vi "对称性单.vi"(11 "XY图":cluster{dbl[], dbl[]}[](graph)) -> (3 "对称性":dbl)   [LabVIEW 2020]
uses:
  <vilib>/Analysis/NI_AAL_Geometry.lvlib
panel:
  out "右":dbl
  out "左":dbl
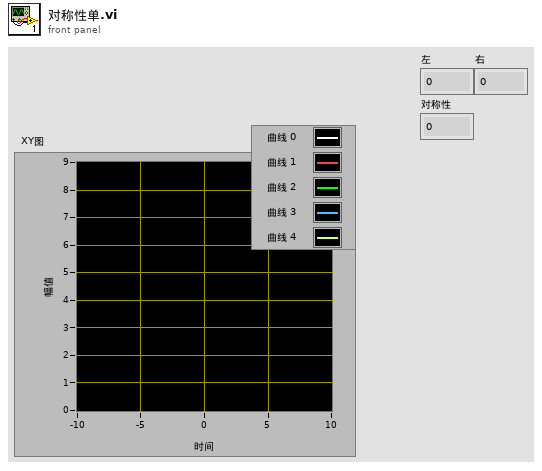
[diagram p1: front panel]
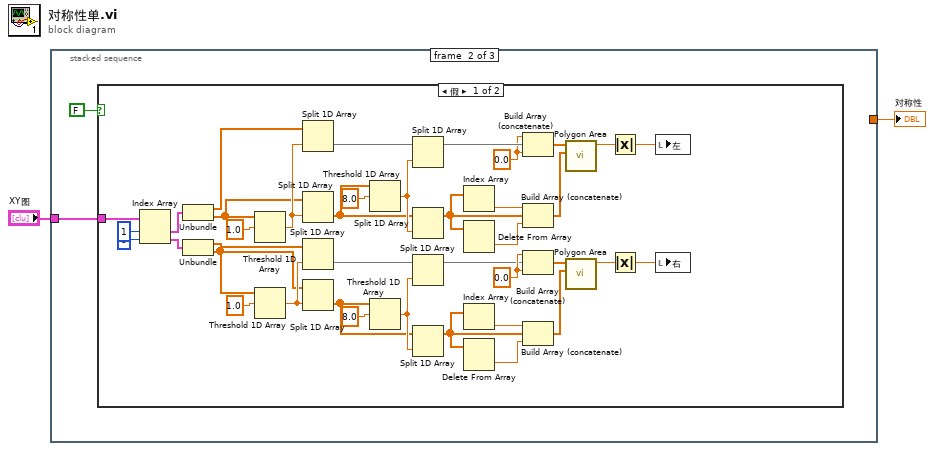
[diagram p0: block diagram]
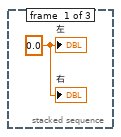
[diagram p2: hidden frame]
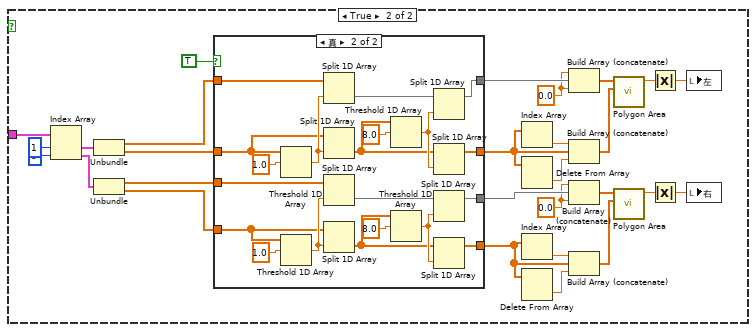
[diagram p3: hidden frame]
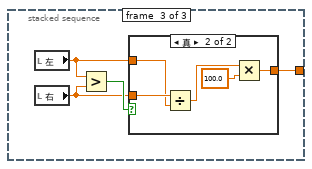
[diagram p5: hidden frame]
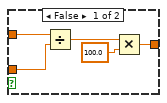
[diagram p6: hidden frame]
diagram:
  n1 = stacked-sequence {
    tunnel: "XY图" -> [_ w4 _]
    tunnel: [_ _ w97] -> w2
    frame #0 {
      w3 = 0.0 ("左")
      "左" <- w3
      "右" <- w3
    }
    frame #1 {
      n2 = case shown="假" FALSE {
        tunnel: w4 -> [w39 w49]
        frame False {
          w13 = 0.0
          w21 = 0.0
          n3 = Index Array(array=w39, index #1=1 ("索引"), index #2=3 ("索引")) -> (element #1=w40:cluster{dbl[], dbl[]}, element #2=w8:cluster{dbl[], dbl[]})
          n4 = Unbundle(w40) -> (w37:dbl[], w31:dbl[])
          n5 = Unbundle(w8) -> (w32:dbl[], w33:dbl[])
          n6 = Threshold 1D Array(2:1.0 ("阈值y"), 3:w31) -> (0:w36:dbl)  [unwired: 1 in]
          n7 = Threshold 1D Array(2:1.0 ("阈值y"), 3:w33) -> (0:w35:dbl)  [unwired: 1 in]
          n8 = Split 1D Array(array=w37, index=w36) -> (second subarray=w28:dbl[])  [unwired: 1 out]
          n9 = Split 1D Array(array=w31, index=w36) -> (second subarray=w27:dbl[])  [unwired: 1 out]
          n10 = Split 1D Array(array=w32, index=w35) -> (second subarray=w24:dbl[])  [unwired: 1 out]
          n11 = Split 1D Array(array=w33, index=w35) -> (second subarray=w23:dbl[])  [unwired: 1 out]
          n12 = Threshold 1D Array(2:8.0 ("阈值y"), 3:w27) -> (0:w30:dbl)  [unwired: 1 in]
          n13 = Threshold 1D Array(2:8.0 ("阈值y"), 3:w23) -> (0:w25:dbl)  [unwired: 1 in]
          n14 = Split 1D Array(array=w28, index=w30) -> (first subarray=w22:dbl[])  [unwired: 1 out]
          n15 = Split 1D Array(array=w27, index=w30) -> (first subarray=w19:dbl[])  [unwired: 1 out]
          n16 = Split 1D Array(array=w24, index=w25) -> (first subarray=w11:dbl[])  [unwired: 1 out]
          n17 = Split 1D Array(array=w23, index=w25) -> (first subarray=w12:dbl[])  [unwired: 1 out]
          n18 = Index Array(array=w19) -> (element=w20:dbl)  [unwired: 1 in]
          n19 = Delete From Array(array=w19) -> (deleted portion=w18:dbl)  [unwired: 2 in, 1 out]
          n20 = Index Array(array=w12) -> (element=w14:dbl)  [unwired: 1 in]
          n21 = Delete From Array(array=w12) -> (deleted portion=w15:dbl)  [unwired: 2 in, 1 out]
          n22 = Build Array (concatenate)(w21, w22, w21) -> (w17:dbl[])
          n23 = Build Array (concatenate)(w20, w19, w18) -> (w16:dbl[])
          n24 = Build Array (concatenate)(w13, w11, w13) -> (w10:dbl[])
          n25 = Build Array (concatenate)(w14, w12, w15) -> (w9:dbl[])
          n26 = call <vilib>:"Polygon Area.vi"("Y"=w16, "X"=w17) -> ("signed area"=w41:dbl)  [unwired: 8 in, 1 out]
          n27 = call <vilib>:"Polygon Area.vi"("Y"=w9, "X"=w10) -> ("signed area"=w43:dbl)  [unwired: 8 in, 1 out]
          n28 = Absolute Value(x=w41) -> (abs(x)=w42:dbl)
          n29 = Absolute Value(x=w43) -> (abs(x)=w44:dbl)
          n30 = local write "左"(w42) -> ()
          n31 = local write "右"(w44) -> ()
        }
        frame True {
          w51 = 0.0
          w50 = 0.0
          n32 = Index Array(array=w49, index #1=1 ("索引"), index #2=3 ("索引")) -> (element #1=w68:cluster{dbl[], dbl[]}, element #2=w47:cluster{dbl[], dbl[]})
          n33 = Unbundle(w68) -> (w67:dbl[], w64:dbl[])
          n34 = Unbundle(w47) -> (w65:dbl[], w66:dbl[])
          n35 = case shown="真" TRUE {
            tunnel: w67 -> [w76 w96]
            tunnel: w66 -> [w73 w93]
            tunnel: w65 -> [w74 w92]
            tunnel: w64 -> [w75 w91]
            tunnel: [w76 w84] -> w63
            tunnel: [w75 w83] -> w61
            tunnel: [w73 w82] -> w55
            tunnel: [w74 w81] -> w54
            frame False {
            }
            frame True {
              n36 = Threshold 1D Array(2:1.0 ("阈值y"), 3:w91) -> (0:w95:dbl)  [unwired: 1 in]
              n37 = Threshold 1D Array(2:1.0 ("阈值y"), 3:w93) -> (0:w94:dbl)  [unwired: 1 in]
              n38 = Split 1D Array(array=w96, index=w95) -> (second subarray=w89:dbl[])  [unwired: 1 out]
              n39 = Split 1D Array(array=w91, index=w95) -> (second subarray=w88:dbl[])  [unwired: 1 out]
              n40 = Split 1D Array(array=w92, index=w94) -> (second subarray=w86:dbl[])  [unwired: 1 out]
              n41 = Split 1D Array(array=w93, index=w94) -> (second subarray=w85:dbl[])  [unwired: 1 out]
              n42 = Threshold 1D Array(2:8.0 ("阈值y"), 3:w88) -> (0:w90:dbl)  [unwired: 1 in]
              n43 = Threshold 1D Array(2:8.0 ("阈值y"), 3:w85) -> (0:w87:dbl)  [unwired: 1 in]
              n44 = Split 1D Array(array=w89, index=w90) -> (first subarray=w84:dbl[])  [unwired: 1 out]
              n45 = Split 1D Array(array=w88, index=w90) -> (first subarray=w83:dbl[])  [unwired: 1 out]
              n46 = Split 1D Array(array=w86, index=w87) -> (first subarray=w81:dbl[])  [unwired: 1 out]
              n47 = Split 1D Array(array=w85, index=w87) -> (first subarray=w82:dbl[])  [unwired: 1 out]
            }
          }
          n48 = Index Array(array=w61) -> (element=w62:dbl)  [unwired: 1 in]
          n49 = Delete From Array(array=w61) -> (deleted portion=w60:dbl)  [unwired: 2 in, 1 out]
          n50 = Index Array(array=w55) -> (element=w56:dbl)  [unwired: 1 in]
          n51 = Delete From Array(array=w55) -> (deleted portion=w57:dbl)  [unwired: 2 in, 1 out]
          n52 = Build Array (concatenate)(w50, w63, w50) -> (w59:dbl[])
          n53 = Build Array (concatenate)(w62, w61, w60) -> (w58:dbl[])
          n54 = Build Array (concatenate)(w51, w54, w51) -> (w53:dbl[])
          n55 = Build Array (concatenate)(w56, w55, w57) -> (w52:dbl[])
          n56 = call <vilib>:"Polygon Area.vi"("Y"=w58, "X"=w59) -> ("signed area"=w69:dbl)  [unwired: 8 in, 1 out]
          n57 = call <vilib>:"Polygon Area.vi"("Y"=w52, "X"=w53) -> ("signed area"=w71:dbl)  [unwired: 8 in, 1 out]
          n58 = Absolute Value(x=w69) -> (abs(x)=w70:dbl)
          n59 = Absolute Value(x=w71) -> (abs(x)=w72:dbl)
          n60 = local write "左"(w70) -> ()
          n61 = local write "右"(w72) -> ()
        }
      }
    }
    frame #2 {
      n62 = local read "左"() -> (w98:dbl)
      n63 = local read "右"() -> (w99:dbl)
      n64 = Greater?(x=w98, y=w99) -> (0:w100:bool)
      n65 = case shown="真" w100 {
        tunnel: w99 -> [w104 w110]
        tunnel: w98 -> [w105 w109]
        tunnel: [w101 w107] -> w97
        frame False {
          n66 = Divide(x=w105, y=w104) -> (x/y=w103:dbl)
          n67 = Multiply(x=w103, y=100.0) -> (x*y=w101:dbl)
        }
        frame True {
          n68 = Divide(x=w110, y=w109) -> (x/y=w108:dbl)
          n69 = Multiply(x=w108, y=100.0) -> (x*y=w107:dbl)
        }
      }
    }
  }
  "对称性" <- w2
